vi "Stop Core.vi"(10 "final error code":i32, 11 "Task Actor in":refnum<class "Task Actor.lvclass">) -> (3 "Task Actor out":refnum<class "Task Actor.lvclass">)   [LabVIEW 2023, in "Task Actor.lvlib" / "Task Actor.lvclass"]
doc: "(<B>Filename</B>: Actor Framework.lvlib:Actor.lvclass:Stop Core.vi)\n\nDefines what the actor does before it stops. Use the <B>final error code</B> input to determine whether the actor shut down in response to an error.\n\nBy default, this method passes the Stop message along to all auto-stop nested actors. A descendant class may override this method to define additional behavior, such as shutting down any processes the actor initiated in its override of the Actor Core method."
uses:
  Task Actor.lvclass
  Task Actor.lvclass/Task Actor.ctl
  Task Base/Task Base.lvclass/Task Base.ctl
  <vilib>/ActorFramework/Actor/Actor.lvclass
  Task Base/Task Base.lvclass
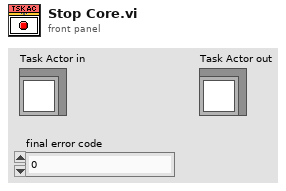
[diagram p1: front panel]
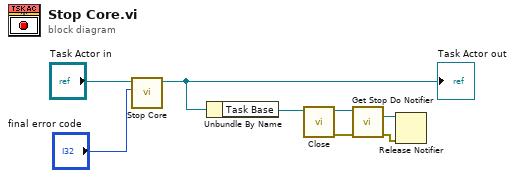
[diagram p0: block diagram]
diagram:
  n1 = call-parent "Stop Core.vi"("final error code"="final error code", "Actor in"="Task Actor in") -> ("Actor out"=w6:refnum<class "Task Actor.lvclass">)  [unwired: 9 in]
  "Task Actor out" <- w6
  n2 = Unbundle By Name(w6) -> ("Task Base"=w5:refnum<class "Task Base.lvclass">)
  n3 = call-dynamic "Close.vi"("Task Base in"=w5) -> ("error out"=w4:errorcluster, "Task Base out"=w3:refnum<class "Task Base.lvclass">)  [unwired: 9 in]
  n4 = call "Get Stop Do Notifier.vi"("error in (no error)"=w4, "Task Base in"=w3) -> ("error out"=w2:errorcluster, "Stop Do"=w1:refnum<notifier>)  [unwired: 7 in, 1 out]
  n5 = Release Notifier(notifier=w1, error in (no error)=w2) -> ()  [unwired: 1 in, 3 out]
